vi "Tektronix AFG 3000 Series Standard Waveform.vi"() -> ()   [LabVIEW 2018]
doc: "Demonstrates how to generate a standard waveform."
uses:
  <instrlib>/Tektronix AFG 3000 Series/Tektronix AFG 3000 Series.lvlib
panel:
  in  "Channel (0: Channel 1)":u16(ring) items=["Channel 1", "Channel 2"]
  in  "DC Offset (0.00 V)":dbl
  in  "Amplitude (1 Vpp)":dbl=1.0
  in  "Waveform Function (0: Sine)":u16(ring) items=["Sine", "Square", "Pulse", "Ramp", "Noise", "DC", "Sin(x)/x", "Gaussian", "Lorentz", "Exponential Rise", "Exponential Decay", "Haversine"]
  in  "Frequency (1000 Hz)":dbl=1000.0
  in  "VISA resource name":refnum<visa-resource-name>
  # "(c) 2006-2019 National Instruments.  ALL RIGHTS RESERVED."
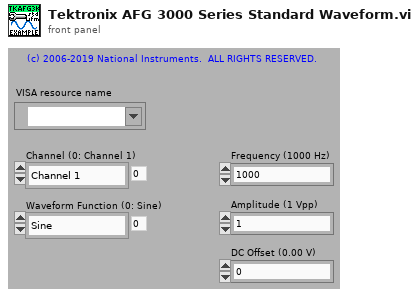
[diagram p1: front panel]
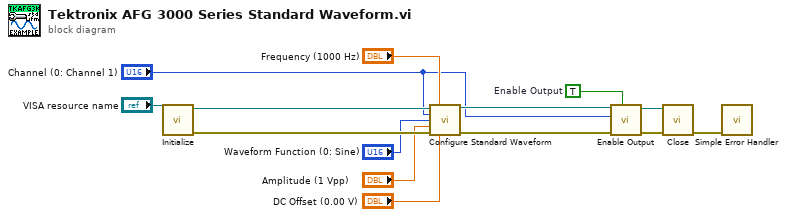
[diagram p0: block diagram]
diagram:
  w2 = TRUE  # Enable Output
  n1 = call <instrlib>:"Initialize.vi"("VISA resource name"="VISA resource name") -> ("error out"=w13:errorcluster, "VISA resource name out"=w14:refnum<visa-resource-name>)  [unwired: 9 in]
  n2 = call <instrlib>:"Configure Standard Waveform.vi"("VISA resource name"=w14, "Frequency (1000 Hz)"="Frequency (1000 Hz)", "Channel (0: Channel 1)"="Channel (0: Channel 1)", "Waveform Function (0: Sine)"="Waveform Function (0: Sine)", "Amplitude (1 Vpp)"="Amplitude (1 Vpp)", "error in (no error)"=w13, "DC Offset (0.00 V)"="DC Offset (0.00 V)") -> ("VISA resource name out"=w11:refnum<visa-resource-name>, "error out"=w10:errorcluster)  [unwired: 7 in]
  n3 = call <instrlib>:"Enable Output.vi"("Enable Output (T: Enable)"=w2, "error in (no error)"=w10, "Channel (0: Channel 1)"="Channel (0: Channel 1)", "VISA resource name"=w11) -> ("error out"=w8:errorcluster, "VISA resource name out"=w9:refnum<visa-resource-name>)  [unwired: 6 in]
  n4 = call <instrlib>:"Close.vi"("error in (no error)"=w8, "VISA resource name"=w9) -> ("error out"=w12:errorcluster)  [unwired: 9 in]
  n5 = call <vilib>:"Simple Error Handler.vi"("error in (no error)"=w12) -> ()  [unwired: 4 in, 5 out]
